vi "Status SRQ.vi"(8 "error in (no error)":errorcluster, 10 "Address (0)":i32, 11 "VISA resource name":refnum<visa-resource-name>) -> (0 "error out":errorcluster, 1 "SRQ (Bool [8])":bool[](array[boolean]), 2 "SRQ (U8)":u8 format="%.0b", 3 "VISA resource name out":refnum<visa-resource-name>)   [LabVIEW 2021, in "Environment Chamber.lvlib" / "Climatic Chamber.lvlib"]
doc: "<b>Interrupt Information.</b>\n\nReturns the state of the SRQ (Service Request) status.\n\nSRQ1: Not used\nSRQ2: When an alarm occurs on the chamber, 1 is set.\nSRQ3: When a single-step operation ends in remote program mode, 1 is set.\nSRQ4: When the state transitions from power off to operation, or vice versa, 1 isset.\nSRQ5: Not used\nSRQ6: Not used\nSRQ7: Reserved with the SRQ function for GPIB communication\nSRQ8: Not used"
uses:
  Climatic Chamber.lvlib
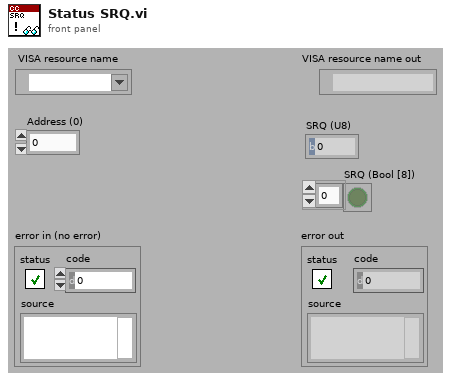
[diagram p1: front panel]
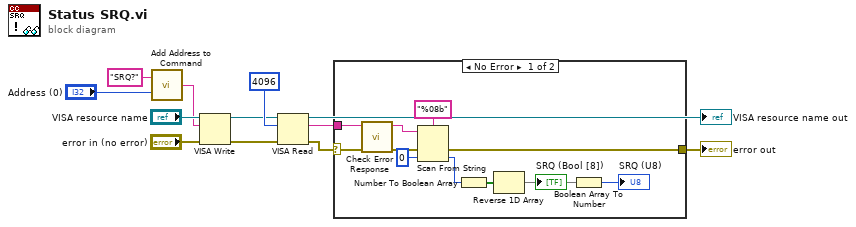
[diagram p0: block diagram]
diagram:
  n1 = call "Add Address to Command.vi"("Address (0)"="Address (0)", "Command"="SRQ?") -> ("Command OUT"=w5:string)
  n2 = VISA Write(VISA resource name="VISA resource name", write buffer=w5, error in (no error)="error in (no error)") -> (VISA resource name out=w9:refnum<visa-resource-name>, error out=w8:errorcluster)  [unwired: 1 out]
  n3 = VISA Read(VISA resource name=w9, byte count=u32 4096, error in (no error)=w8) -> (VISA resource name out=→"VISA resource name out":refnum<visa-resource-name>, read buffer=w3:string, error out=w4:errorcluster)  [unwired: 1 out]
  n4 = case shown="No Error" w4 {
    selector: w4 -> [w22 w24]
    tunnel: w3 -> [w23 _]
    tunnel: [w19 w24] -> w2
    frame No Error {
      n5 = call "Check Error Response.vi"("error in (no error)"=w22, "read String"=w23) -> ("error out"=w20:errorcluster, "String out"=w18:string)  [unwired: 7 in, 1 out]
      n6 = Scan From String(format string="%08b", input string=w18, error in=w20, default 1=u8 0 ("default value 1")) -> (error out=w19:errorcluster, output 1=w17:u8)  [unwired: 1 in, 2 out]
      n7 = Number To Boolean Array(number=w17) -> (Boolean array=w16:bool[])
      n8 = Reverse 1D Array(array=w16) -> (reversed array=w14:bool[])
      "SRQ (Bool [8])" <- w14
      n9 = Boolean Array To Number(Boolean array=w14) -> (number=→"SRQ (U8)":u8)
    }
    frame Error {
    }
  }
  "error out" <- w2
